vi "Global_Claw_Rotation_Offset.vi"() -> ()   [LabVIEW 2017]
panel:
  out "Offset":dbl
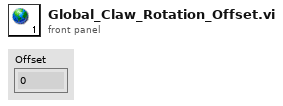
[diagram p1: front panel]
diagram:
